vi "SendFile1.vi"(4 "error in":errorcluster, 6 "Array":T1(array[cluster])) -> (0 "error out":errorcluster, 1 "last ses time":timestamp)   [LabVIEW 2010]
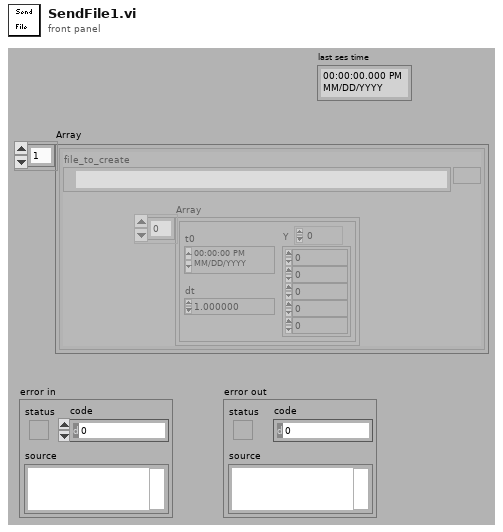
[diagram p1: front panel]
types:
  T1 = cluster{"file_to_create":path, "Array":waveform(i16)[]}[]
  T2 = cluster{i32, "date str":string, "microseconds str":string, "max_values":string[]}
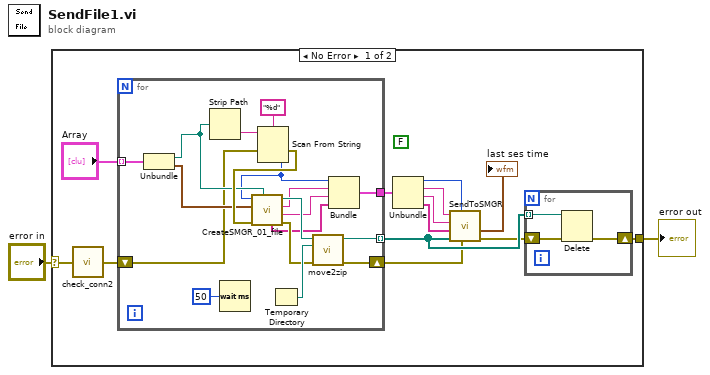
[diagram p0: block diagram]
diagram:
  n1 = case shown="No Error" "error in" {
    selector: "error in" -> [w4 w37]
    tunnel: [w12 w37] -> w2
    frame No Error {
      (unwired) FALSE
      n2 = call "check_conn2.vi"("error IO"=w4) -> ("error out"=w3:errorcluster)
      n3 = for {
        tunnel: "Array" -> [w30] mode=indexing
        tunnel: [w26] -> w14 mode=indexing
        shift-right: [w25] -> w13
        shift-left: w3 -> [w27]
        tunnel: [w21] -> w11
        n4 = Unbundle(w30) -> ("file_to_create"=w29:path, "Array"=w28:waveform(i16)[])
        n5 = Strip Path(path=w29) -> (name=w32:string)  [unwired: 1 out]
        n6 = Wait (ms)(milliseconds to wait=u32 50) -> ()  [unwired: 1 out]
        n7 = Scan From String(format string="%d", input string=w32, error in=w27) -> (error out=w31:errorcluster, output 1=w20:i32)  [unwired: 2 in, 2 out]
        n8 = call "CreateSMGR_01_file.vi"("file path to write"=w29, "error in"=w31, "Waveform Graph"=w28, "meas_point"=w20) -> ("error out"=w34:errorcluster, "microseconds str"=w23:string, "date str"=w24:string, "file path out"=w35:path, "max_values"=w22:string[])  [unwired: 3 in]
        n9 = Temporary Directory() -> (w36:path)
        n10 = call "move2zip.vi"("error in"=w34, "dest dir"=w36, "source path"=w35) -> ("error out"=w25:errorcluster, "zipped path"=w26:path)  [unwired: 3 in]
        n11 = Bundle(w20, "date str"=w24, "microseconds str"=w23, "max_values"=w22) -> (w21:T2)  [unwired: 1 in]
      }
      n12 = Unbundle(w11) -> (w9:i32, "date str"=w6:string, "microseconds str"=w8:string, "max_values"=w5:string[])
      n13 = call "SendToSMGR.vi"("error in"=w13, "meas_point"=w9, "Files"=w14, "max_value_"=w5, "microseconds"=w8, "date"=w6) -> ("error out"=w10:errorcluster, "last ses time"=→"last ses time":timestamp)  [unwired: 1 in, 3 out]
      n14 = for {
        tunnel: w14 -> [w16] mode=indexing
        shift-right: [w17] -> w12
        shift-left: w10 -> [w18]
        n15 = Delete(path (use dialog)=w16, error in=w18) -> (error out=w17:errorcluster)  [unwired: 3 in, 2 out]
      }
    }
    frame Error {
    }
  }
  "error out" <- w2
